vi "PH_BL-Master.PC calc O2 State.vi"(0 "i ref in":refnum<vi>, 2 "O2 Instance":string="N/A", 4 "no link":bool, 5 "error in (no error)":errorcluster) -> (14 "i ref out":refnum<vi>, 19 "error out":errorcluster)   [LabVIEW 2014, in "PH_BL-Master.lvlib"]
doc: "This VI sets the vac state to GUI elements and stores it to own attributes."
uses:
  PH_BL-Master.lvlib
  PH_Basics/PH_StatusHandler/PH_StatusHandler.Status.ctl
  PH_Basics/PH_StatusHandler/PH_StatusHandler.lvlib
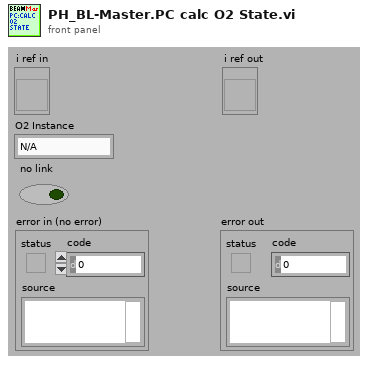
[diagram p1: front panel]
types:
  T1 = typedef "PH_BL-Master.lvlib/PH_BL-Master.i attribute.ctl" = cluster{"Remote controlled":bool, "Boolean Condition Service Subscriber":refnum<vi>[], "Picture Condition Service Subscriber":refnum<vi>[], "R2S":cluster{"GUI Ref":refnum<vi>, "State":bool}, "Vacua":cluster{"GUI Ref":refnum<vi>, "Limit":dbl, "Curr Value":dbl, "in range":bool}[], "O2 Inspection":cluster{"GUI Ref":refnum<vi>, "Concentration":dbl, "State":T2}[], "Boolean Status Service Subscriber":cluster{"GUI Ref":refnum<vi>, "Status":T2, "no Link?":bool, "Status Subscriber Class":T3}[], "Picture Status Service Subscriber":cluster{"GUI Ref":refnum<vi>, "Status":T2, "no Link?":bool, "Status Subscriber Class":T3}[], "6P 4Q Service Subscriber":cluster{"GUI Ref":refnum<vi>, "Selector":T4, "no Link?":bool}[], "Index of latest 6P 4Q changing Instance":i32, "Index of latest Picture Status changing Instance":i32, "Index of latest Boolean Status changing Instance":i32, "Vision ID on same Node":string, "Start Phase over?":bool, "GUI Ref Delete":refnum<vi>}
  T2 = typedef "PH_StatusHandler.lvlib/PH_StatusHandler.Status.ctl" = i16
  T3 = typedef "PH_BL-Master.lvlib/PH_BL-Master.Status Subscriber Class.ctl" = enum16{"unknown", "Switch", "BB", "6P Switch", "Switch GUI", "Switch and 6P State", "Force Sensor"}
  T4 = typedef "PH_4_Pos_Selector.lvlib/PH_4_Pos_Selector.Position Selector.ctl" = u16
  T5 = cluster{"GUI Ref":refnum<vi>, "Concentration":dbl, "State":T2}[]
  T6 = cluster{"GUI Ref":refnum<vi>, "Concentration":dbl, "State":T2}
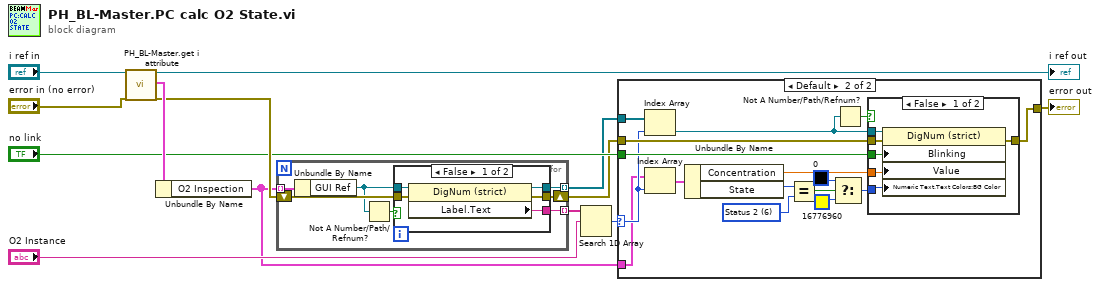
[diagram p0: block diagram]
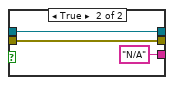
[diagram p2: hidden frame]
diagram:
  n1 = call "PH_BL-Master.get i attribute.vi"("i ref in"="i ref in", "error in (no error)"="error in (no error)") -> ("i ref out"=→"i ref out":refnum<vi>, "i attribute"=w13:T1, "error out"=w12:errorcluster)  [unwired: 15 in]
  n2 = Unbundle By Name(w13) -> ("O2 Inspection"=w2:T5)
  n3 = for {
    tunnel: [w20] -> w7 mode=indexing
    shift-right: [w18] -> w6
    shift-left: w12 -> [w19]
    tunnel: w2 -> [w16] mode=indexing
    tunnel: [w14] -> w1 mode=indexing
    n4 = Unbundle By Name(w16) -> ("GUI Ref"=w15:refnum<vi>)
    n5 = Not A Number/Path/Refnum?(number/path/refnum=w15) -> (NaN/Path/Refnum?=w17:bool)
    n6 = case shown="False" w17 {
      tunnel: w15 -> [w25 w26]
      tunnel: [w24 "N/A" ("Label.Text")] -> w20
      tunnel: w19 -> [w23 w28]
      tunnel: [w22 w28] -> w18
      tunnel: [w21 w26] -> w14
      frame False {
        n7 = property class="DigNum (strict)"(reference=w25, error in=w23) -> (reference out=w21:refnum<vi>, error out=w22:errorcluster, "Label.Text"=w24:string)
      }
      frame True {
      }
    }
  }
  n8 = Search 1D Array(1D array=w7, element="O2 Instance") -> (index of element=w5:i32)  [unwired: 1 in]
  n9 = case shown="Default" w5 {
    selector: w5 -> [_ w35]
    tunnel: w6 -> [w29 w45]
    tunnel: [w29 w44] -> w3
    tunnel: "no link" -> [_ w39]
    tunnel: w2 -> [_ w32]
    tunnel: w1 -> [_ w31]
    frame -1 {
    }
    frame Default {
      w36 = T2 6 items=["no info", "off/false/out", "on/true/in", "Failure", "Alarm", "Status 1", "Status 2", "Status 3"] ("State")
      n10 = Index Array(array=w31, index=w35) -> (element=w30:refnum<vi>)
      n11 = Index Array(array=w32, index=w35) -> (element=w38:T6)
      n12 = Unbundle By Name(w38) -> ("Concentration"=w34:dbl, "State"=w37:T2)
      n13 = Equal?(x=w37, y=w36) -> (x = y?=w33:bool)
      n14 = Select(t=u32 0 ("Color Box"), s=w33, f=u32 16776960 ("Color Box")) -> (s? t:f=w41:u32)
      n15 = Not A Number/Path/Refnum?(number/path/refnum=w30) -> (NaN/Path/Refnum?=w40:bool)
      n16 = case shown="False" w40 {
        tunnel: w30 -> [w51 _]
        tunnel: w45 -> [w50 w52]
        tunnel: [w49 w52] -> w44
        tunnel: w34 -> [w48 _]
        tunnel: w41 -> [w47 _]
        tunnel: w39 -> [w46 _]
        frame False {
          n17 = property class="DigNum (strict)"(reference=w51, error in=w50, "Blinking"=w46, "Value"=w48, "Numeric Text.Text Colors:BG Color"=w47) -> (error out=w49:errorcluster)  [unwired: 1 out]
        }
        frame True {
        }
      }
    }
  }
  "error out" <- w3
